vi "Host-FIXParser-TestHarness.vi"() -> ()   [LabVIEW 2020]
uses:
  <vilib>/rvi/interface/RandomDataEmulation/nirviRandomDataOpen.vi
  <vilib>/rvi/interface/RandomDataEmulation/nirviRandomDataDMAMethods.vi
  <vilib>/rvi/interface/RandomDataEmulation/nirviRandomDataClose.vi
  <vilib>/rvi/interface/nirviOpenFPGA/nirviOpenFPGA.xnode
  FIXParser-TestHarness-Typedef.ctl
  FPGA/Tests/Fpga-FIXParser-TestHarness.vi
  <vilib>/rvi/interface/nirviMethod/nirviMethod.xnode
  <vilib>/rvi/interface/nirviCloseFPGA/nirviCloseFPGA.xnode
panel:
  out "Array":T1(array[cluster])
  out "Raw Data Length":i32
  out "Raw Data":u64[][](array[numeric]) format="%.0x"
  out "error out":errorcluster
  in  "file path (use dialog)":path=path "E:/work/git/fpganow/FIXParser/SamplesMessages/TestBed.dat"
  in  "error in":errorcluster
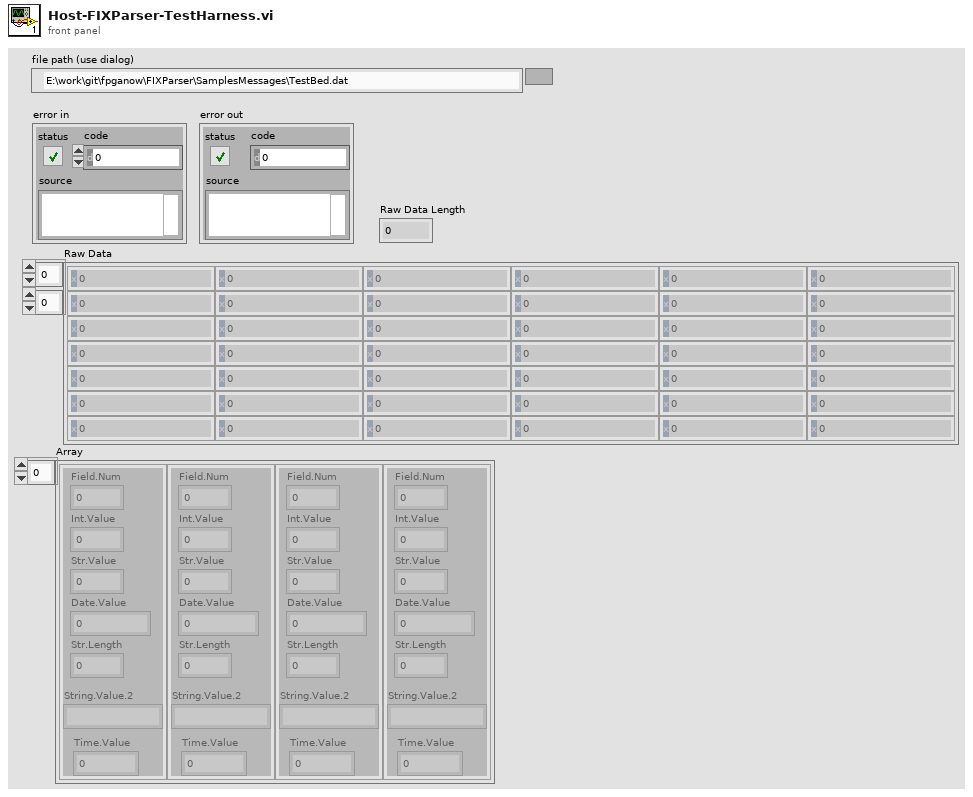
[diagram p1: front panel]
types:
  T1 = cluster{"Field.Num":u16, "Int.Value":u16, "Str.Value":u64, "Date.Value":u64, "Str.Length":u32, "String.Value.2":string, "Time.Value":u64}[]
  T2 = typedef "FIXParser-TestHarness-Typedef.ctl" = refnum<k20>
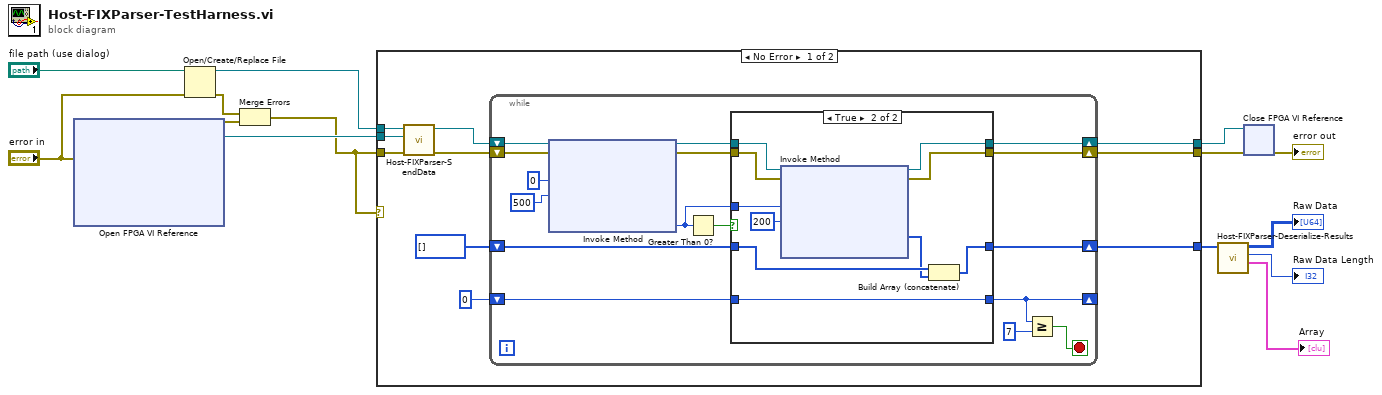
[diagram p0: block diagram]
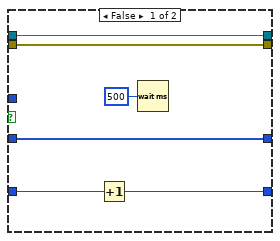
[diagram p2: hidden frame]
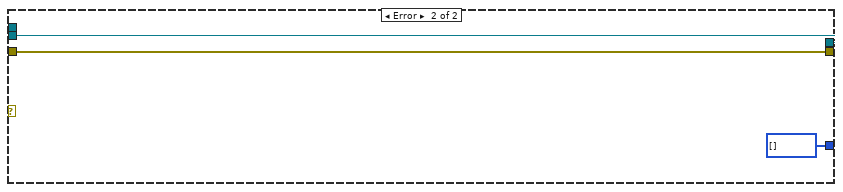
[diagram p3: hidden frame]
diagram:
  n1 = xnode "Open FPGA VI Reference"("error in"="error in") -> ("FPGA VI Reference Out"=w14:T2, "error out"=w9:errorcluster)  [unwired: 1 in]
  n2 = Open/Create/Replace File(file path (use dialog)="file path (use dialog)", error in="error in") -> (refnum out=w12:refnum<file>, error out=w10:errorcluster)  [unwired: 4 in, 1 out]
  n3 = Merge Errors(w10, w9) -> (w8:errorcluster)
  n4 = case shown="No Error" w8 {
    tunnel: w14 -> [w24 w58]
    tunnel: [w19 w59] -> w6
    tunnel: w12 -> [w21 _]
    tunnel: w8 -> [w20 w59]
    tunnel: [w18 w58] -> w5
    tunnel: [w15 u64[] [] ("Data 2")] -> w4
    frame No Error {
      n5 = call "Host-FIXParser-SendData.vi"("error in\n(no error)"=w20, "FPGA VI Reference In"=w24, "Byte Stream\nFile in"=w21) -> ("error out"=w22:errorcluster, "FPGA VI Reference Out"=w23:T2)  [unwired: 7 in]
      n6 = while {
        shift-right: [w29] -> w15
        shift-left: u64[] [] ("Data 2") -> [w30]
        shift-right: [w32] -> w18
        shift-left: w23 -> [w40]
        shift-right: [w31] -> w19
        shift-left: w22 -> [w33]
        shift-right: [w27] -> _
        shift-left: 0 -> [w28]
        stop <- w25 stop-if-true
        n7 = xnode "Invoke Method"("FPGA VI Reference In"=w40, "error in"=w33, "Number of Elements"=u32 0, "Timeout (ms)"=500) -> ("FPGA VI Reference Out"=w35:T2, "error out"=w34:errorcluster, "Elements Remaining"=w36:u32)  [unwired: 1 out]
        n8 = Greater Than 0?(x=w36) -> (x > 0?=w37:bool)
        n9 = case shown="True" w37 {
          tunnel: w36 -> [_ w56]
          tunnel: w35 -> [w46 w54]
          tunnel: w34 -> [w45 w53]
          tunnel: [w46 w52] -> w32
          tunnel: [w45 w51] -> w31
          tunnel: w30 -> [w44 w50]
          tunnel: [w44 w48] -> w29
          tunnel: [w42 w47] -> w27
          tunnel: w28 -> [w43 w47]
          frame False {
            n10 = Increment(x=w43) -> (x+1=w42:i32)
            n11 = Wait (ms)(milliseconds to wait=u32 500) -> ()  [unwired: 1 out]
          }
          frame True {
            n12 = xnode "Invoke Method"("FPGA VI Reference In"=w54, "error in"=w53, "Number of Elements"=w56, "Timeout (ms)"=200) -> ("FPGA VI Reference Out"=w52:T2, "error out"=w51:errorcluster, "Data"=w49:u64[])  [unwired: 1 out]
            n13 = Build Array (concatenate)(w50, w49) -> (w48:u64[])
          }
        }
        n14 = Greater Or Equal?(x=w27, y=7) -> (x >= y?=w25:bool)
      }
    }
    frame Error {
    }
  }
  n15 = call "Host-FIXParser-Deserialize-Results.vi"("Data in"=w4) -> ("Array"=→"Array":T1, "Raw Data Length"=→"Raw Data Length":i32, "Raw Data"=→"Raw Data":u64[][])  [unwired: 8 in]
  n16 = xnode "Close FPGA VI Reference"("FPGA VI Reference In"=w5, "error in"=w6) -> ("error out"=→"error out":errorcluster)
